vi "Try Match Response.vi"(8 "error in":errorcluster, 10 "ICAN CC Frame":refnum<class "ICAN CC Frame.lvclass">, 11 "Upload Transfer in":refnum<class "Upload Transfer.lvclass">) -> (0 "error out":errorcluster, 2 "Match":bool, 3 "SDO Transfer out":refnum<class "SDO Transfer.lvclass">)   [LabVIEW 2020, in "CANopen.lvlib" / "SDO Manager.lvlib" / "Upload Transfer.lvclass"]
uses:
  Upload Transfer.lvclass
  D:/git/CANopen-LabVIEW/source/SDO/SDO Manager/SDO Transfer/SDO Transfer.lvclass
  SDO Transfer/SDO Transfer.lvclass
  HAL/Source/Interfaces/ICAN CC Frame/ICAN CC Frame.lvclass
  D:/git/HAL/Source/Interfaces/IMessage/IMessage.lvclass
  SDO Transfer/SDO Transfer.lvclass/SDO Transfer.ctl
  CANopen Message/CANopen Message.lvclass
  SDO Transfer/SDO abort code.ctl
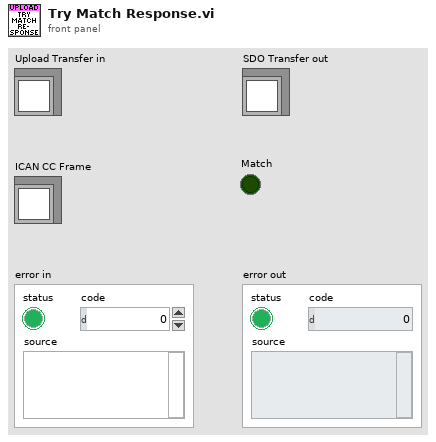
[diagram p1: front panel]
types:
  T1 = typedef "CANopen.lvlib/SDO Manager.lvlib/SDO Transfer.lvclass/SDO abort code.ctl" = u32
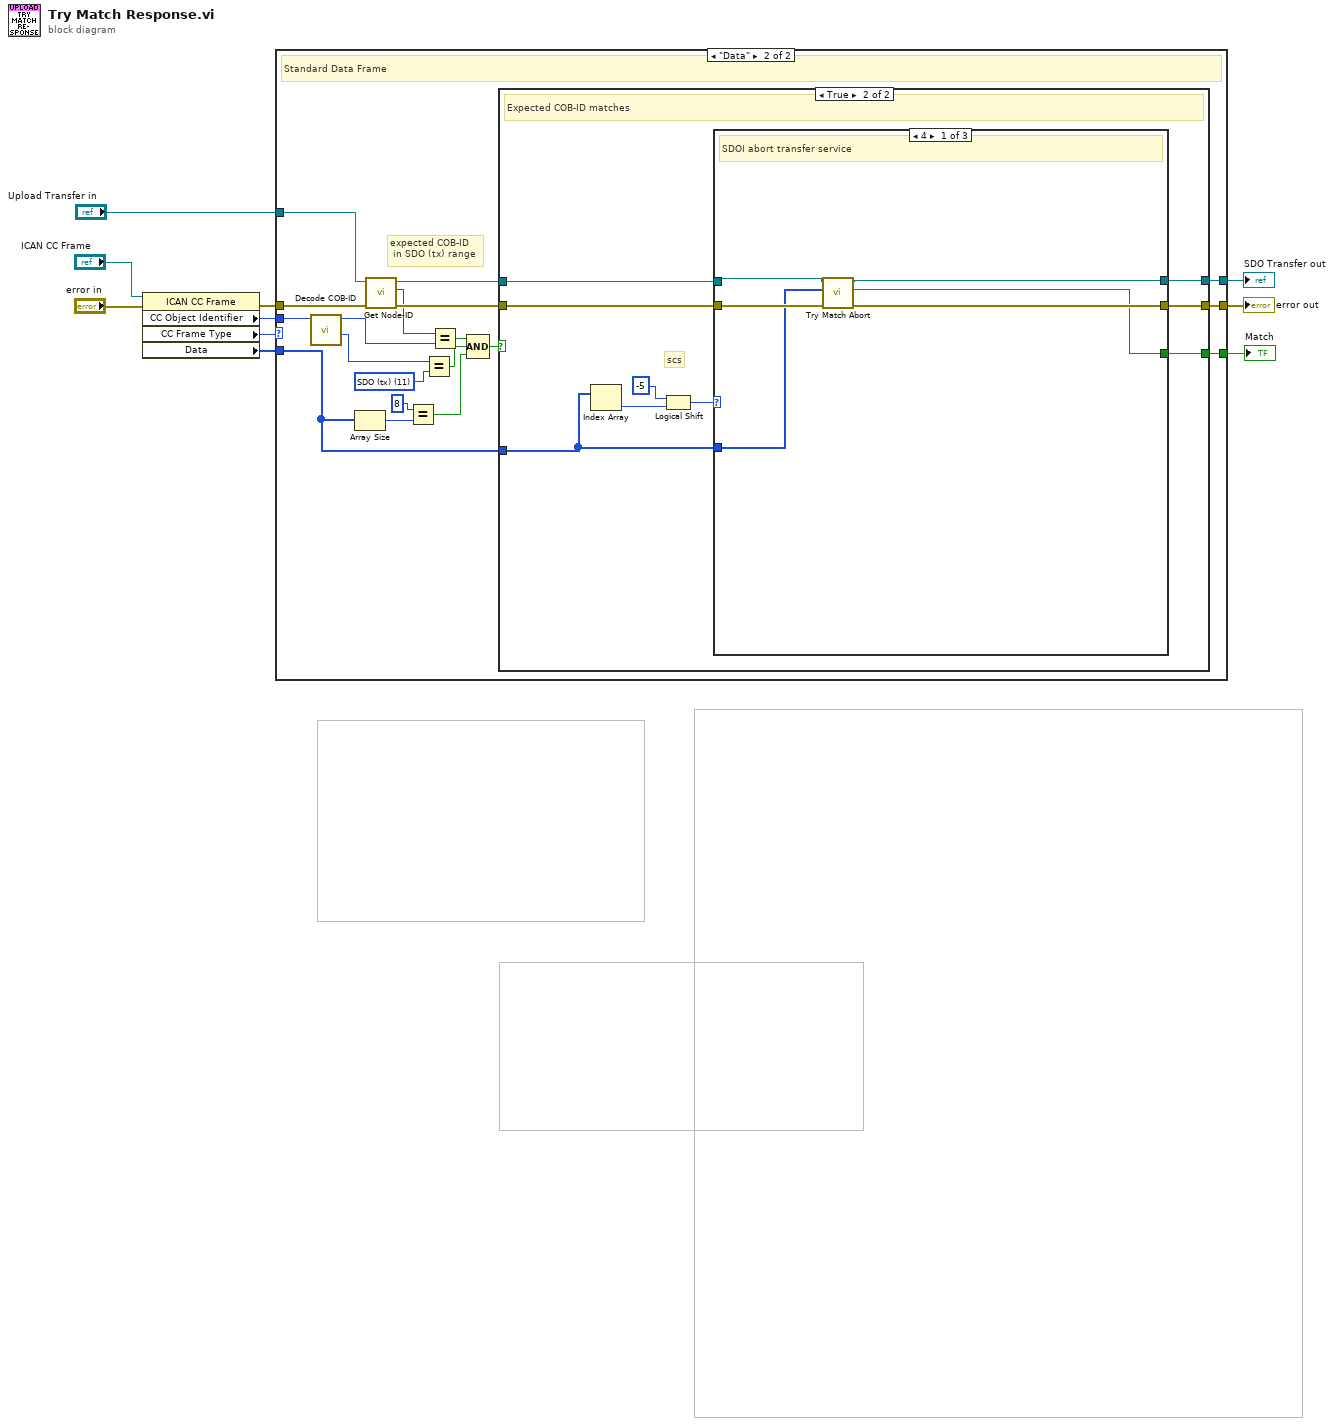
[diagram p0: block diagram]
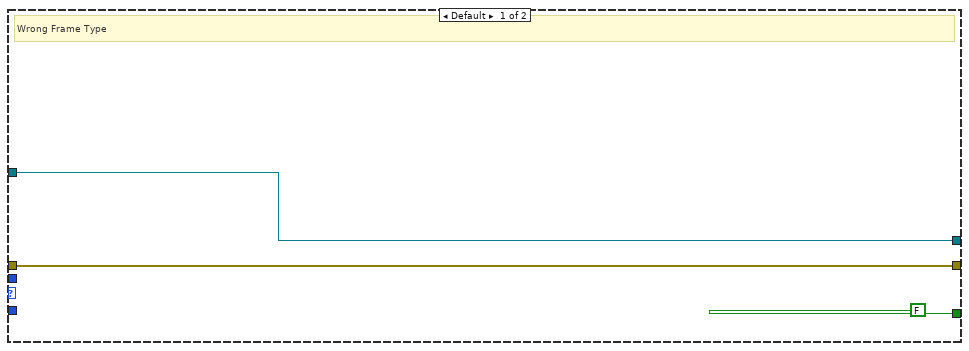
[diagram p2: hidden frame]
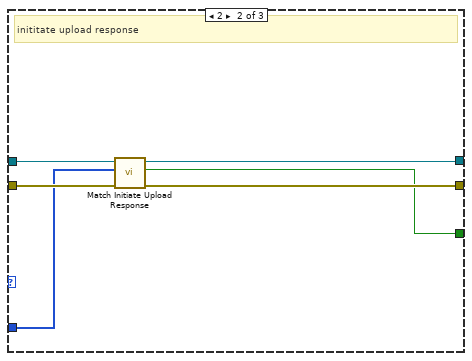
[diagram p4: hidden frame]
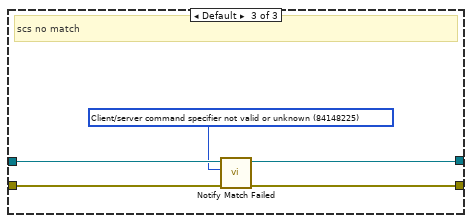
[diagram p5: hidden frame]
diagram:
  n1 = property class="ICAN CC Frame"(reference="ICAN CC Frame", error in="error in") -> (error out=w8:errorcluster, "CC Object Identifier"=w3:u32, "CC Frame Type"=w1:enum8{"Data", "Remote", "Error", "Overload"}, "Data"=w2:u8[])  [unwired: 1 out]
  n2 = case shown="\"Data\"" w1 {
    tunnel: w8 -> [w12 w32]
    tunnel: "Upload Transfer in" -> [w11 w31]
    tunnel: [w11 w28] -> w6
    tunnel: [w12 w27] -> w5
    tunnel: [FALSE w26] -> w4
    tunnel: w3 -> [_ w25]
    tunnel: w2 -> [_ w14]
    frame Default {
      # "Wrong Frame Type"
    }
    frame "Data" {
      w22 = u8 11 items=["NMT"=0, "EMCY/SYNC"=1, "TIME"=2, "PDO1 (tx)"=3, "PDO1 (rx)"=4, "PDO2 (tx)"=5, "PDO2 (rx)"=6, "PDO3 (tx)"=7, "PDO3 (rx)"=8, "PDO4 (tx)"=9, "PDO4 (rx)"=10, "SDO (tx)"=11, "SDO (rx)"=12, "NMT error control"=14] ("Function Code")
      # "expected COB-ID\n in SDO (tx) range"
      # "Standard Data Frame"
      n3 = call "Decode COB-ID.vi"("COD-ID"=w25) -> ("Function Code"=w21:u8, "Node-ID"=w24:u8)  [unwired: 9 in]
      n4 = Array Size(array=w14) -> (size(s)=w20:i32)
      n5 = call "Get Node-ID.vi"("error in"=w32, "SDO Transfer in"=w31) -> ("error out"=w29:errorcluster, "Node-ID"=w23:u8, "SDO Transfer out"=w30:refnum<class "Upload Transfer.lvclass">)  [unwired: 7 in]
      n6 = Equal?(x=8, y=w20) -> (x = y?=w15:bool)
      n7 = Equal?(x=w21, y=w22) -> (x = y?=w16:bool)
      n8 = Equal?(x=w23, y=w24) -> (x = y?=w17:bool)
      n9 = Compound Arithmetic op=AND(w17, w16, w15) -> (w18:bool)
      n10 = case shown="True" w18 {
        tunnel: w30 -> [w34 w42]
        tunnel: w29 -> [w33 w41]
        tunnel: [w34 w38] -> w28
        tunnel: [w33 w39] -> w27
        tunnel: w14 -> [_ w35]
        tunnel: [_ w37] -> w26
        frame False {
        }
        frame True {
          # "scs"
          # "Expected COB-ID matches"
          n11 = Index Array(array=w35) -> (element=w36:u8)  [unwired: 1 in]
          n12 = Logical Shift(y=i16 -5, x=w36) -> (x << y=w40:u8)
          n13 = case shown="4" w40 {
            tunnel: w42 -> [w48 w53 w57]
            tunnel: w41 -> [w49 w55 w60]
            tunnel: [w45 w52 w58] -> w38
            tunnel: [w46 w54 w59] -> w39
            tunnel: [w44 w51 _] -> w37
            tunnel: w35 -> [w47 w50 _]
            frame 4 {
              # "SDOI abort transfer service"
              n14 = call "Try Match Abort.vi"("error in"=w49, "Data"=w47, "SDO Transfer in"=w48) -> ("error out"=w46:errorcluster, "Success"=w44:bool, "SDO Transfer out"=w45:refnum<class "Upload Transfer.lvclass">)  [unwired: 6 in]
            }
            frame 2 {
              # "inititate upload response"
              n15 = call "Match Initiate Upload Response.vi"("error in"=w55, "Frame Data"=w50, "SDO Transfer in"=w53) -> ("error out"=w54:errorcluster, "Match"=w51:bool, "SDO Transfer out"=w52:refnum<class "SDO Transfer.lvclass">)  [unwired: 6 in]
            }
            frame Default {
              w56 = T1 84148225 items=["Toggle bit not allowed"=84082688, "SDO protocol timed out"=84148224, "Client/server command specifier not valid or unknown"=84148225, "Invalid block size (block mode only)"=84148226, "Invalid sequence number (block mode only)"=84148227, "CRC error (block mode only)"=84148228, "Out of memory"=84148229, "Attempt to read a write only object"=100728833, "Attempt to write a read only object"=100728834, "Object does not exist in the object dictionary"=100794368, "Object cannot be mapped to the PDO"=100925505, "The number and length of the objects to be mapped would exceed PDO length"=100925506, "General parameter incompatibility reason"=100925507, "General internal incompatibility in the device"=100925511, "Access failed due to an hardware error"=101056512, "Data type does not match, length of service parameter does not match"=101122064, "Data type does not match, length of service parameter too high"=101122066, "Data type does not match, length of service parameter too low"=101122067, "Sub-index does not exist"=101253137, "Invalid value for parameter (download only)"=101253168, "Value of parameter written too high (download only)"=101253169, "Value of parameter written too low (download only)"=101253170, "Maximum value is less than minimum value"=101253174, "Resource not available: SDO connection"=101318691, "General error"=134217728, "Data cannot be transferred or stored to the application"=134217760, "Data cannot be transferred or stored to the application because of local control"=134217761, "Data cannot be transferred or stored to the application because of the present device stable"=134217762, "Object dictionary dynamic generation fails or no object dictionary is present (e.g. object dictionary is generated from file and generation fails because of an file error)"=134217763, "No data available"=134217764] ("SDO abort code")
              # "scs no match"
              n16 = call "Notify Match Failed.vi"("error in"=w60, "SDO abort code"=w56, "SDO Transfer in"=w57) -> ("error out"=w59:errorcluster, "SDO Transfer out"=w58:refnum<class "Upload Transfer.lvclass">)  [unwired: 7 in]
            }
          }
        }
      }
    }
  }
  "SDO Transfer out" <- w6
  "error out" <- w5
  "Match" <- w4
